vi "CheckAllPages.vi"() -> ()   [LabVIEW 2012]
panel:
  out "Array":T1(array[cluster])
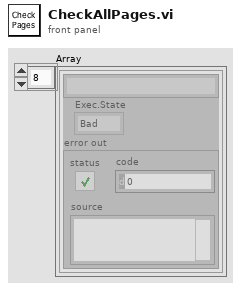
[diagram p1: front panel]
types:
  T1 = cluster{string, "Exec.State":enum32{"Bad", "Idle", "Run top level", "Running"}, "error out":errorcluster}[]
  T2 = enum32{"Bad", "Idle", "Run top level", "Running"}
  T3 = cluster{string, "Exec.State":enum32{"Bad", "Idle", "Run top level", "Running"}, "error out":errorcluster}
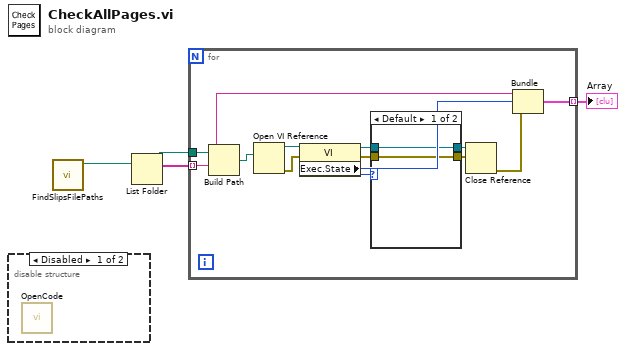
[diagram p0: block diagram]
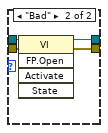
[diagram p3: hidden frame]
diagram:
  n1 = disable-structure shown="Disabled" {
    frame Disabled {
      n2 = call "OpenCode.vi"() -> ()  [unwired: 4 in]
    }
    frame Enabled {
    }
  }
  n3 = call "FindSlipsFilePaths.vi"() -> ("Slides"=w4:path)  [unwired: 2 in, 4 out]
  n4 = List Folder(path=w4) -> (path out=w2:path, filenames=w3:string[])  [unwired: 3 in, 2 out]
  n5 = for {
    tunnel: w3 -> [w12] mode=indexing
    tunnel: w2 -> [w16]
    tunnel: [w10] -> w1 mode=indexing
    n6 = Build Path(base path=w16, name or relative path=w12) -> (appended path=w15:path)
    n7 = Open VI Reference(vi path=w15) -> (vi reference=w14:refnum<vi>, error out=w13:errorcluster)  [unwired: 5 in]
    n8 = property class="VI"(reference=w14, error in=w13) -> (reference out=w9:refnum<vi>, error out=w8:errorcluster, "Exec.State"=w5:T2)
    n9 = case shown="Default" w5 {
      tunnel: w9 -> [w18 w22]
      tunnel: w8 -> [w17 w21]
      tunnel: [w17 w20] -> w7
      tunnel: [w18 w19] -> w6
      frame Default {
      }
      frame "Bad" {
        n10 = invoke class="VI" method="FP.Open"(reference=w22, error in=w21) -> (reference out=w19:refnum<vi>, error out=w20:errorcluster)  [unwired: 3 in, 3 out]
      }
    }
    n11 = Close Reference(reference=w6, error in (no error)=w7) -> (error out=w11:errorcluster)
    n12 = Bundle(w12, "Exec.State"=w5, "error out"=w11) -> (w10:T3)  [unwired: 1 in]
  }
  "Array" <- w1
